vi "Field To Robot Centric.vi"(10 "IMU Value (offset)":dbl, 11 "Translation Joystick":cluster{dbl, dbl}) -> (2 "Robot Centric Vector":cluster{dbl, dbl}, 3 "Wrapped IMU (radians)":dbl)   [LabVIEW 2020]
doc: "Takes in the translation x and y coordinates of the robot, assuming it is field centric, and converts it to polar coordinates. Using the IMU value, it subtracts that from the current heading. Then it converts back to rectangular coordinates which is the new Robot centric coordinates."
uses:
  <vilib>/Analysis/coordinate.llb/Angle Units.ctl
  <vilib>/Analysis/coordinate.llb/Angle Range (Degree).ctl
  <vilib>/Analysis/coordinate.llb/Wrap Angle (scalar).vi
  <vilib>/Analysis/NI_AAL_Angle.lvlib
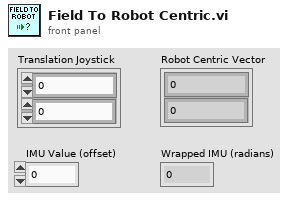
[diagram p1: front panel]
types:
  T1 = typedef "NI_AAL_Angle.lvlib/Angle Range (Degree).ctl" = u16
  T2 = typedef "NI_AAL_Angle.lvlib/Angle Units.ctl" = i32
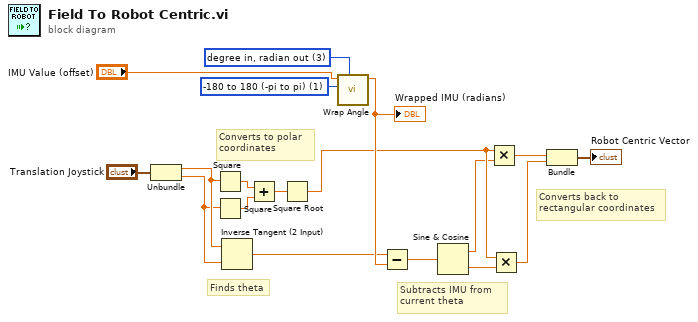
[diagram p0: block diagram]
diagram:
  w17 = T1 1 items=["none", "-180 to 180 (-pi to pi)", "0 to 360 (0 to 2pi)"] ("angle range")
  w18 = T2 3 items=["radian in, radian out", "radian in, degree out", "degree in, degree out", "degree in, radian out"] ("angle units")
  # "Converts back to \nrectangular coordinates"
  # "Subtracts IMU from \ncurrent theta"
  # "Finds theta"
  # "Converts to polar \ncoordinates"
  n1 = Unbundle("Translation Joystick") -> (w2:dbl, w1:dbl)
  n2 = Square(x=w2) -> (x^2=w15:dbl)
  n3 = Square(x=w1) -> (x^2=w14:dbl)
  n4 = Inverse Tangent (2 Input)(1:w1, 2:w2) -> (0:w11:dbl)
  n5 = Add(x=w15, y=w14) -> (x+y=w13:dbl)
  n6 = Square Root(x=w13) -> (sqrt(x)=w10:dbl)
  n7 = call-poly <vilib>:"Wrap Angle.vi"("angle units"=w18, "angle range"=w17, "angle in"="IMU Value (offset)") -> ("angle out"=w12:dbl)  [unwired: 7 in, 1 out]
  "Wrapped IMU (radians)" <- w12
  n8 = Subtract(x=w11, y=w12) -> (x-y=w6:dbl)
  n9 = Sine & Cosine(0:w6) -> (1:w4:dbl, 2:w5:dbl)
  n10 = Multiply(x=w10, y=w4) -> (x*y=w9:dbl)
  n11 = Multiply(x=w10, y=w5) -> (x*y=w8:dbl)
  n12 = Bundle(w9, w8) -> (→"Robot Centric Vector":cluster{dbl, dbl})  [unwired: 1 in]
